vi "Supported Smart Syntax Representation.vi"(0 "Message Popup in":refnum<class "Arithmetic Operations.lvclass">, 11 "error in (no error)":errorcluster) -> (4 "Message Popup out":refnum<class "Arithmetic Operations.lvclass">, 6 "Smart Syntax Representation List":string[](array[string]), 15 "error out":errorcluster)   [LabVIEW 2016, in "Arithmetic Operations.lvclass"]
uses:
  Arithmetic Operations.lvclass
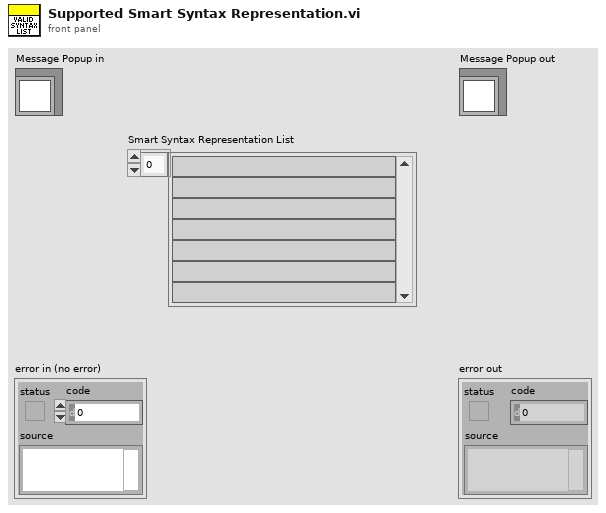
[diagram p1: front panel]
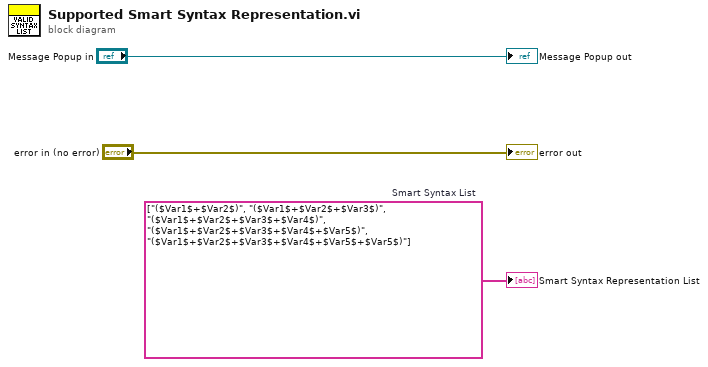
[diagram p0: block diagram]
diagram:
  w1 = string[] ["($Var1$+$Var2$)", "($Var1$+$Var2$+$Var3$)", "($Var1$+$Var2$+$Var3$+$Var4$)", "($Var1$+$Var2$+$Var3$+$Var4$+$Var5$)", "($Var1$+$Var2$+$Var3$+$Var4$+$Var5$+$Var5$)"]  # Smart Syntax List
  "error out" <- "error in (no error)"
  "Message Popup out" <- "Message Popup in"
  "Smart Syntax Representation List" <- w1
